vi "Save path length.vi"(3 "Path Length data":string, 5 "Step":dbl, 7 "Animal Number":dbl, 11 "Path length data":dbl[][](array[numeric])) -> ()   [LabVIEW 2020]
panel:
  out "concatenated string 2":string
  out "Path Length Data":dbl[][](array[numeric])
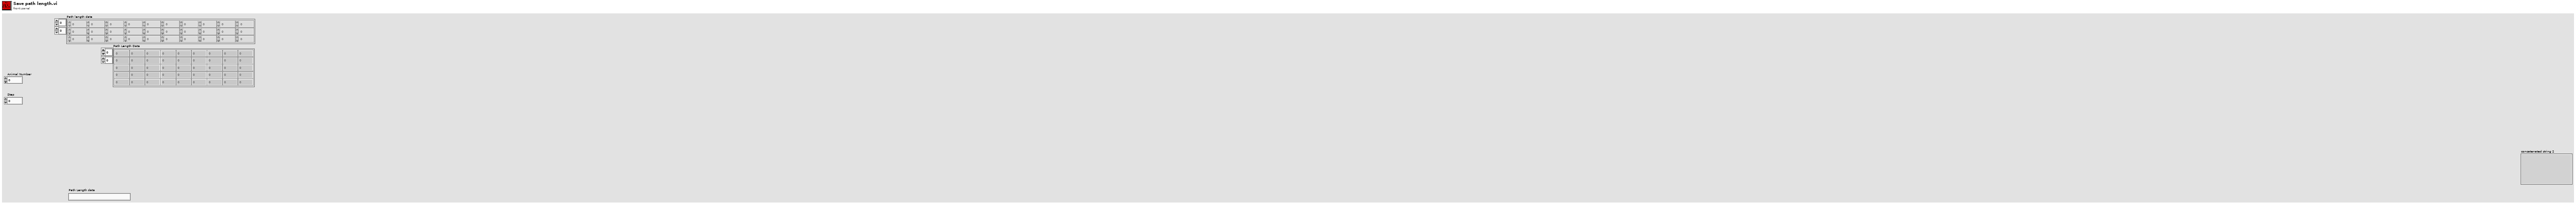
[diagram p1: front panel]
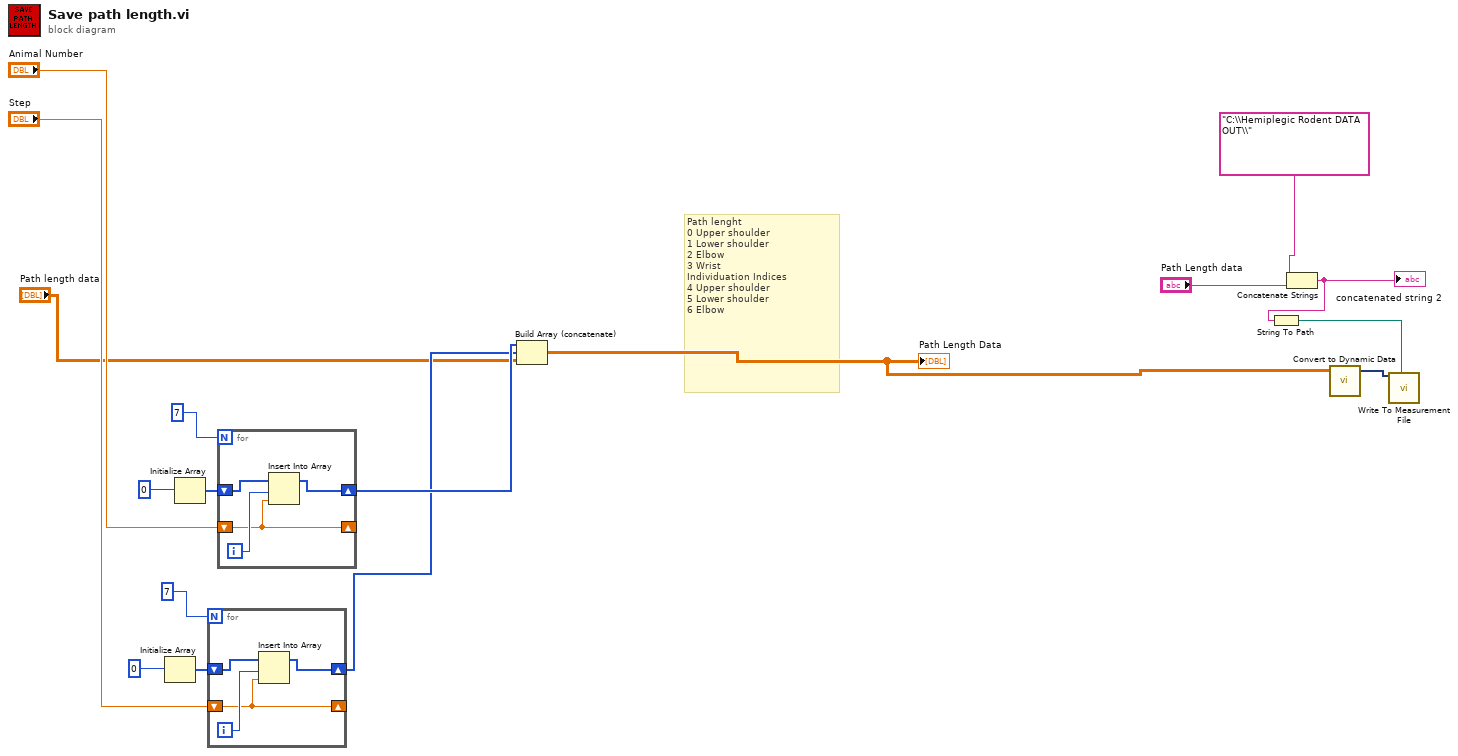
[diagram p0: block diagram]
diagram:
  # "Path lenght\n0 Upper shoulder\n1 Lower shoulder\n2 Elbow\n3 Wrist\nIndividuation Indices\n4 Upper shoulder\n5 Lower shoulder\n6 Elbow"
  n1 = Initialize Array(0) -> (w12:i32[])  [unwired: 1 in]
  n2 = Initialize Array(0) -> (w15:i32[])  [unwired: 1 in]
  n3 = for {
    N: 7 -> [_]
    shift-right: [w19] -> w8
    shift-left: w12 -> [w20]
    shift-right: [w18] -> _
    shift-left: "Step" -> [w18]
    i -> [w21]
    n4 = Insert Into Array(array=w20, index=w21, new element=w18) -> (w19:i32[])
  }
  n5 = for {
    N: 7 -> [_]
    shift-right: [w23] -> w9
    shift-left: w15 -> [w24]
    shift-right: [w22] -> _
    shift-left: "Animal Number" -> [w22]
    i -> [w25]
    n6 = Insert Into Array(array=w24, index=w25, new element=w22) -> (w23:i32[])
  }
  n7 = Build Array (concatenate)(w9, w8, "Path length data") -> (w1:dbl[][])
  "Path Length Data" <- w1
  n8 = Concatenate Strings("C:\\Hemiplegic Rodent DATA OUT\\" ("name"), "Path Length data") -> (w5:string)
  "concatenated string 2" <- w5
  n9 = String To Path(string=w5) -> (path=w3:path)
  n10 = call "Convert to Dynamic Data"("2D Array"=w1) -> ("Dynamic Data Type"=w2:dynamicdata)  [unwired: 3 in]
  n11 = call "Write To Measurement File"("Signals"=w2, "Filename"=w3) -> ()  [unwired: 15 in, 3 out]
